vi "PAQmem_getLatestUnsavedRAM.vi"(8 "error in (no error)":errorcluster, 11 "FAMM in":refnum<class "FAMM.lvclass">) -> (0 "error out":errorcluster, 2 "Data_2_Save":T1(array[cluster]), 3 "FAMM out":refnum<class "FAMM.lvclass">)   [LabVIEW 2020, in "FAMM.lvclass"]
doc: "Get latest memory from FAMM that is not yet saved to the database."
uses:
  FAMM.lvclass
  FAMM.lvclass/FAMM.ctl
  PAQ-memory.lvclass
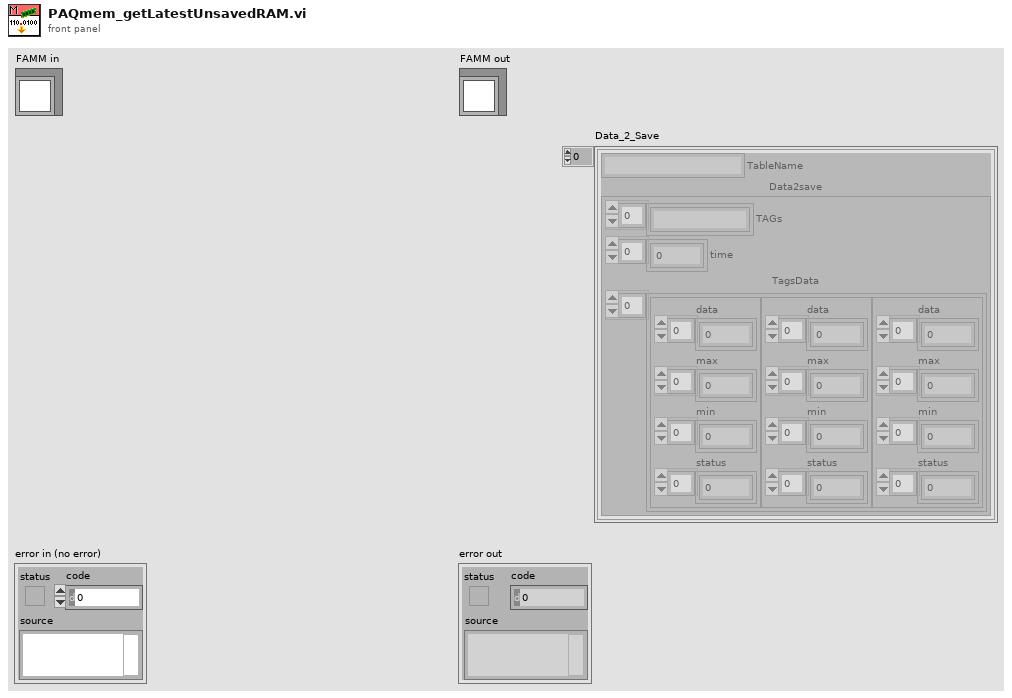
[diagram p1: front panel]
types:
  T1 = cluster{"TableName":string, "Data2save":cluster{"TAGs":string[], "time":dbl[], "TagsData":cluster{"data":dbl[], "max":dbl[], "min":dbl[], "status":u32[]}[]}}[]
  T2 = cluster{"TableName":string, "Data2save":cluster{"TAGs":string[], "time":dbl[], "TagsData":cluster{"data":dbl[], "max":dbl[], "min":dbl[], "status":u32[]}[]}}
  T3 = typedef "FAMM.lvclass/FAMM-attributes.ctl" = cluster{"FAMM_PAQ_Layers":i32, "FAMM_PAQ_resolution":dbl, "PAQ_TAGs":string[], "WAQ_TAGs":string[], "EAQ_TAGs":string[], "All_TAGs":string[], "PAQtagProps":T4[], "WAQtagProps":T4[], "EAQtagProps":T4[], "DBAL_class":refnum<data-value>, "PAQ_memory":refnum<data-value>[], "PAQupdates":timestamp[], "FAMM_Size":cluster{"other":i32, "1day":i32, "1week":i32}, "DatabaseFileExtention":string, "DatabaseSaveRate":dbl, "Database_path":path, "DBAL-Queue":refnum<queue>}
  T4 = typedef "typedef_com_TagProp.ctl" = cluster{"Description":string, "EngUnits":string, "RangeH":dbl, "RangeL":dbl, "Resolution":i32, "Obsolete":bool, "ChangeDate":timestamp, "ChangeSource":string, "ChangeReason":string, "TagFunc":u32}
  T5 = cluster{"TAGs":string[], "time":dbl[], "TagsData":cluster{"data":dbl[], "max":dbl[], "min":dbl[], "status":u32[]}[]}
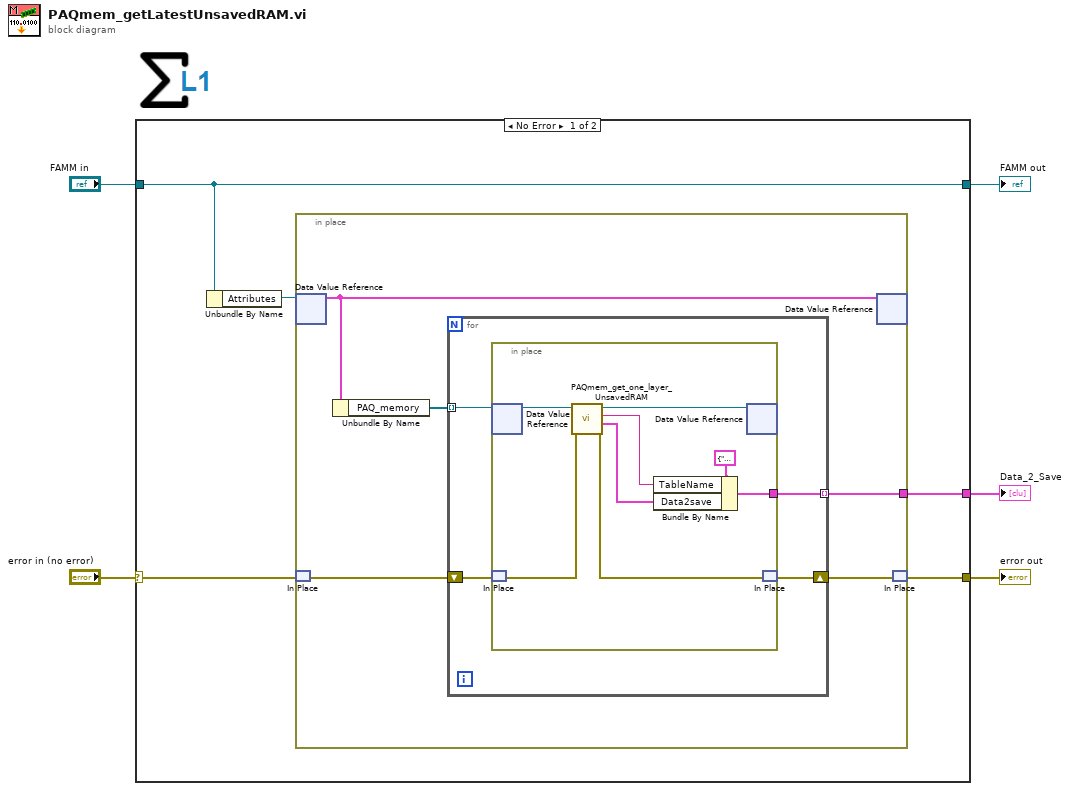
[diagram p0: block diagram]
diagram:
  n1 = case shown="No Error" "error in (no error)" {
    selector: "error in (no error)" -> [w10 w29]
    tunnel: [w9 w29] -> w4
    tunnel: [w7 w28] -> w2
    tunnel: "FAMM in" -> [w7 w28]
    tunnel: [w8 _] -> w1
    frame No Error {
      n2 = Unbundle By Name(w7) -> ("Attributes"=w6:refnum<data-value>)
      n3 = in-place {
        in-place-border: [w11] -> w8
        n4 = in-place-dvr #1(w6) -> (w15:T3)  [unwired: 1 out]
        n5 = in-place-match #2(w10) -> (w13:errorcluster)
        n6 = Unbundle By Name(w15) -> ("PAQ_memory"=w14:refnum<data-value>[])
        n7 = for {
          tunnel: w14 -> [w19] mode=indexing
          shift-right: [w17] -> w12
          shift-left: w13 -> [w18]
          tunnel: [w16] -> w11 mode=indexing
          n8 = in-place {
            in-place-border: [w20] -> w16
            n9 = in-place-dvr #3(w19) -> (w27:refnum<class "PAQ-memory.lvclass">)  [unwired: 1 out]
            n10 = in-place-match #4(w18) -> (w25:errorcluster)
            n11 = call "PAQmem_get_one_layer_UnsavedRAM.vi"("error in (no error)"=w25, "PAQ-memory in"=w27) -> ("error out"=w24:errorcluster, "Data2save"=w21:T5, "TableName"=w22:string, "PAQ-memory out"=w26:refnum<class "PAQ-memory.lvclass">)  [unwired: 6 in]
            n12 = Bundle By Name(cluster=T2 {"TableName"="", "Data2save"={"TAGs"=[], "time"=[], "TagsData"=[]}} ("Unsaved_PAQ_Layer_Portion"), "TableName"=w22, "Data2save"=w21) -> (w20:T2)
            n13 = in-place-dvr #3(w26) -> ()  [unwired: 2 out]
            n14 = in-place-match #4(w24) -> (w17:errorcluster)
          }
        }
        n15 = in-place-dvr #1(w15) -> ()  [unwired: 2 out]
        n16 = in-place-match #2(w12) -> (w9:errorcluster)
      }
    }
    frame Error {
    }
  }
  "error out" <- w4
  "FAMM out" <- w2
  "Data_2_Save" <- w1
